vi "Main X-Y.vi"(0 "Home position X":dbl, 1 "Home position Y":dbl, 3 "Move position Y (# of steps)":dbl, 5 "Move position X (# of steps)":dbl, 7 "Change Home position Y?":bool, 9 "Return Home X":bool, 12 "Return Home Y":bool, 13 "Stop":bool, 14 "Move to Set Position":bool) -> (4 "Get/Acquire RT position X":dbl, 6 "Get/Acquire RT position Y":dbl, 8 "X-axes Motion":dbl(knob) scale=0.0..200.0, 10 "Y-axes Motion":dbl(knob) scale=0.0..200.0)   [LabVIEW 2018]
doc: "X-Y motion control simulator app that demonstrates control of the X-Y stage for a given system hardware"
panel:
  in  "Change Home position X?":bool
  out "System Ready?":bool
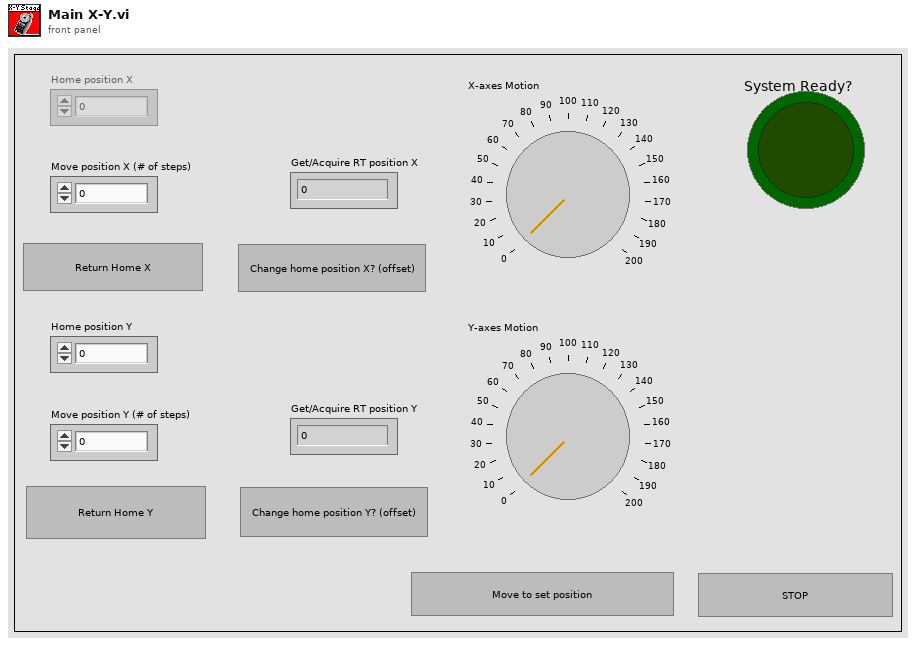
[diagram p1: front panel]
types:
  T1 = enum32{"Invalid", "Standard", "Closed", "Hidden", "Minimized", "Maximized"}
  T2 = enum32{"invalid app kind", "Development System", "Run Time System", "Student Edition", "Embedded LabVIEW", "Evaluation", "Custom"}
  T3 = enum8{"Enabled", "Disabled", "Disabled and Grayed Out"}
  T4 = cluster{"Core":cluster{"Current VI Reference":refnum<vi>, "Close Panel on Exit?":bool}, "System Ready?":bool, string}
  T5 = cluster{"Current VI Reference":refnum<vi>, "Close Panel on Exit?":bool}
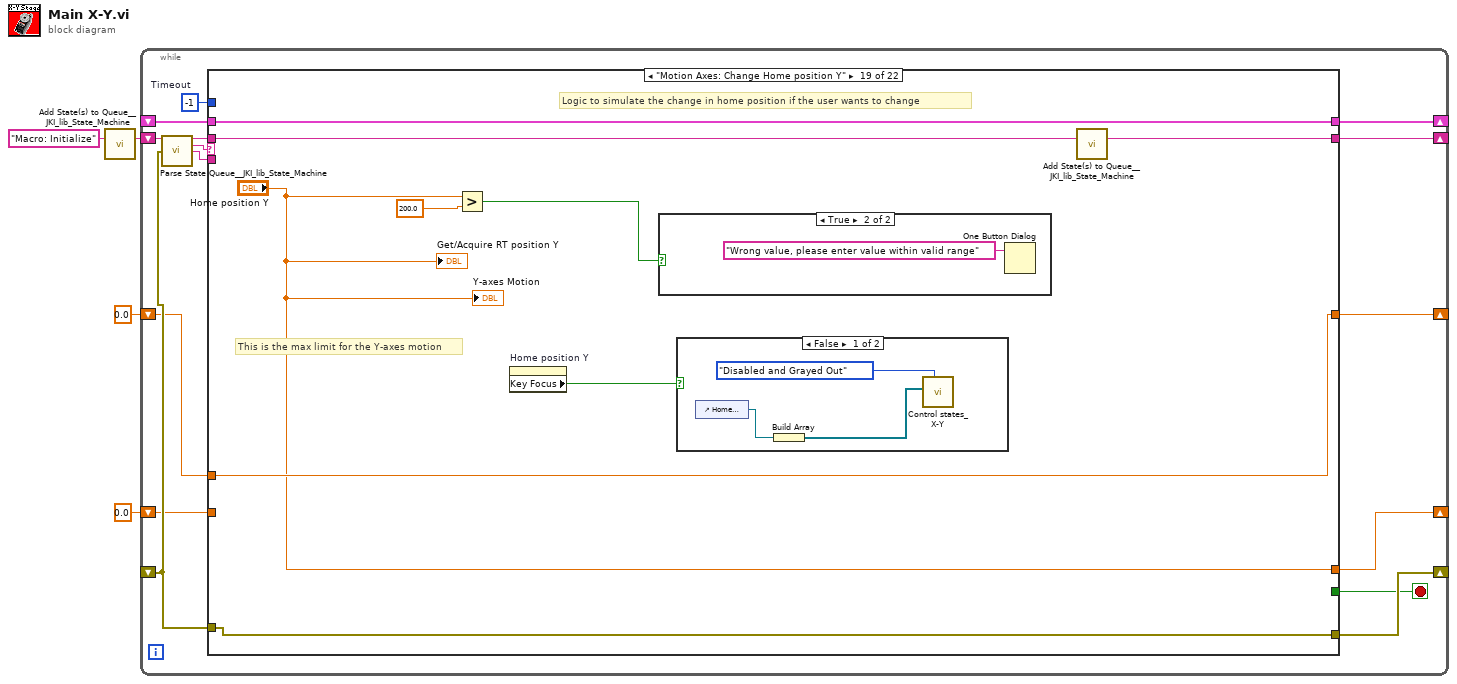
[diagram p0: block diagram]
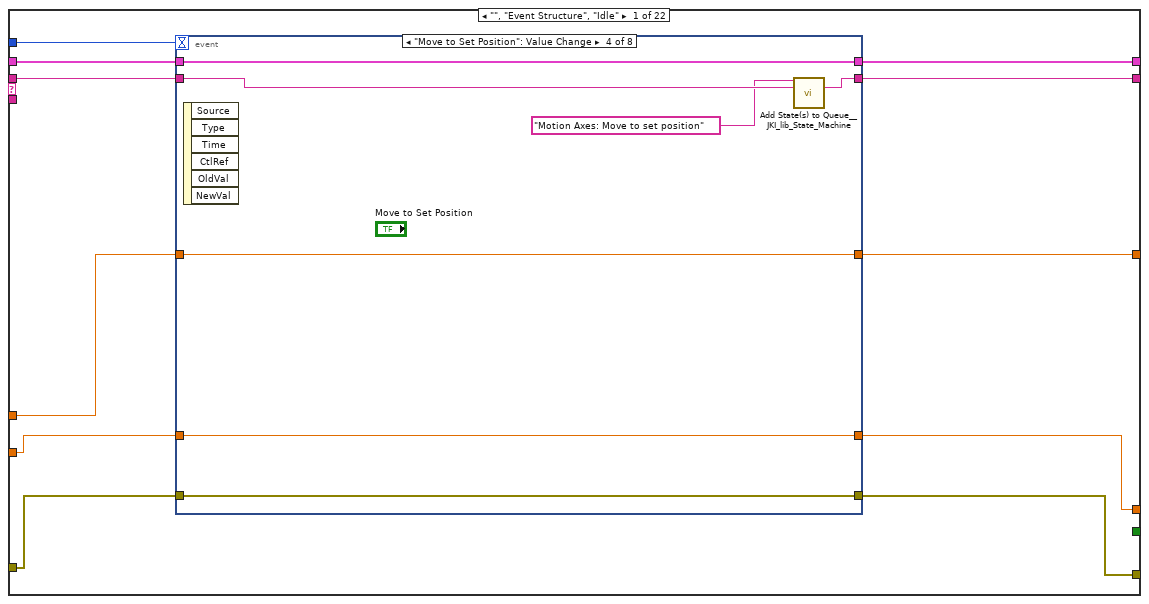
[diagram p2: hidden frame]
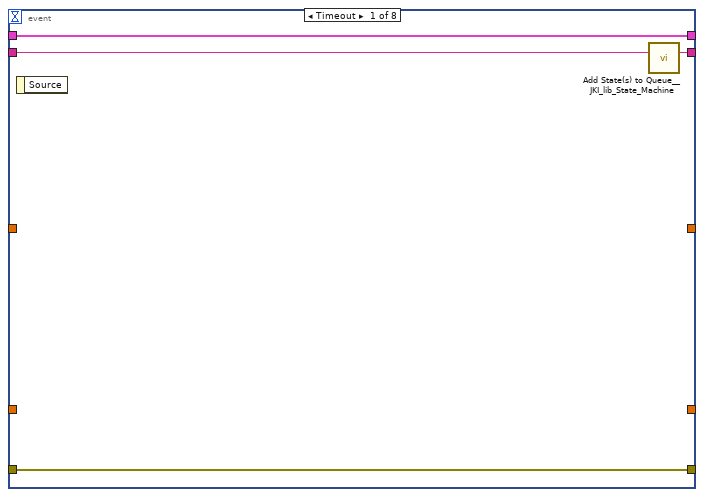
[diagram p3: hidden frame]
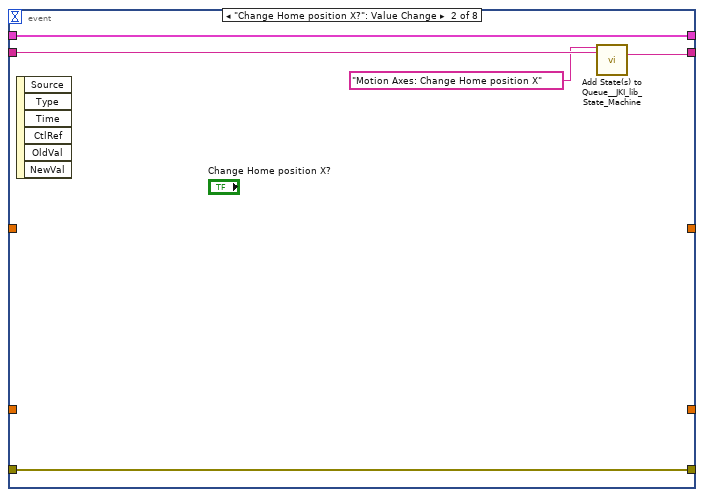
[diagram p4: hidden frame]
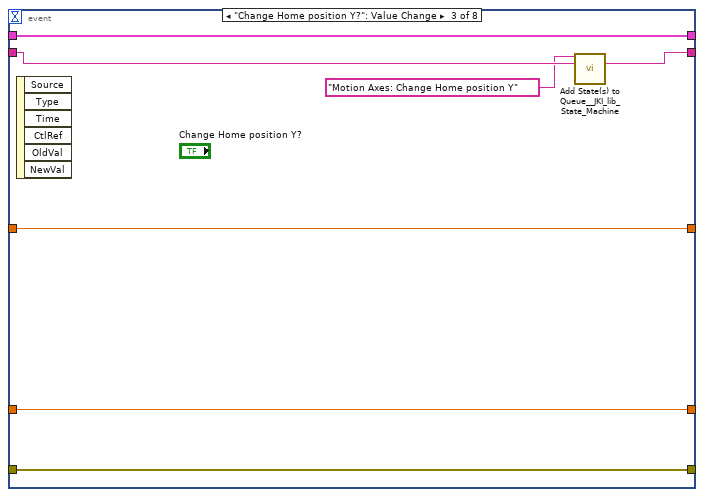
[diagram p5: hidden frame]
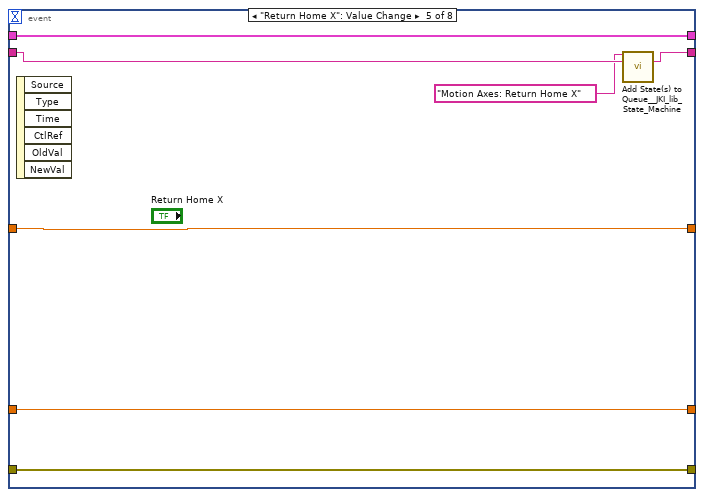
[diagram p6: hidden frame]
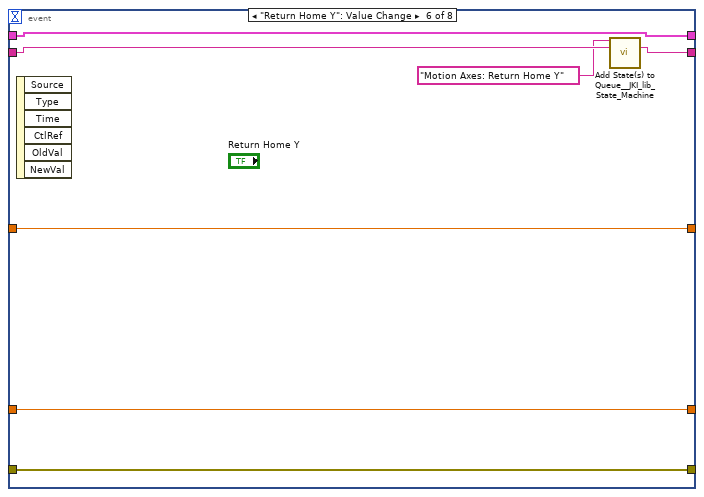
[diagram p7: hidden frame]
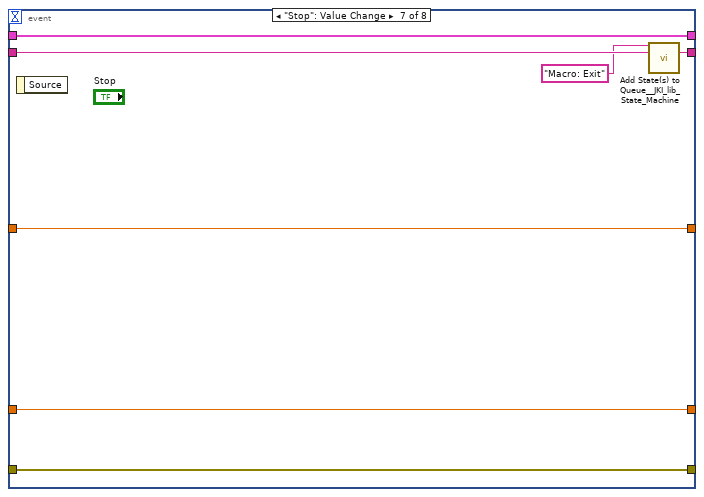
[diagram p8: hidden frame]
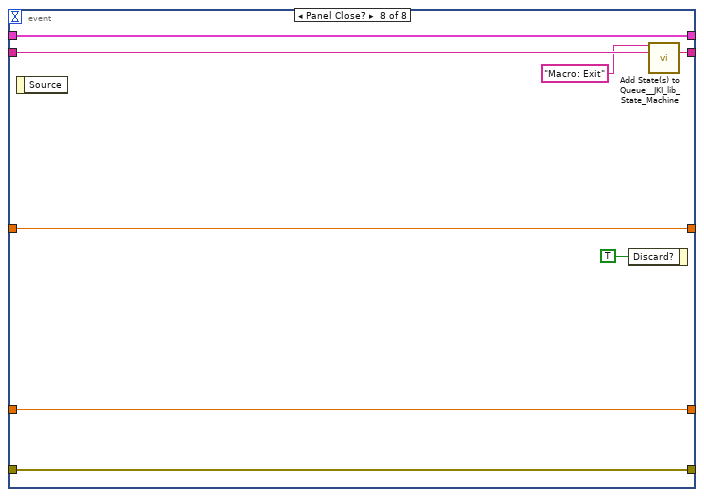
[diagram p9: hidden frame]
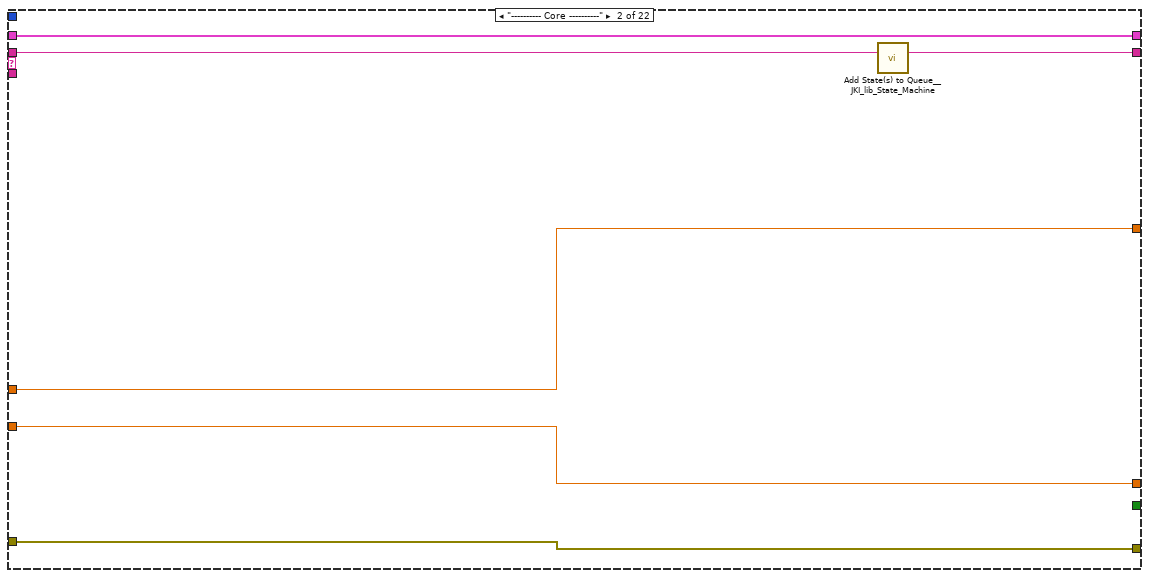
[diagram p10: hidden frame]
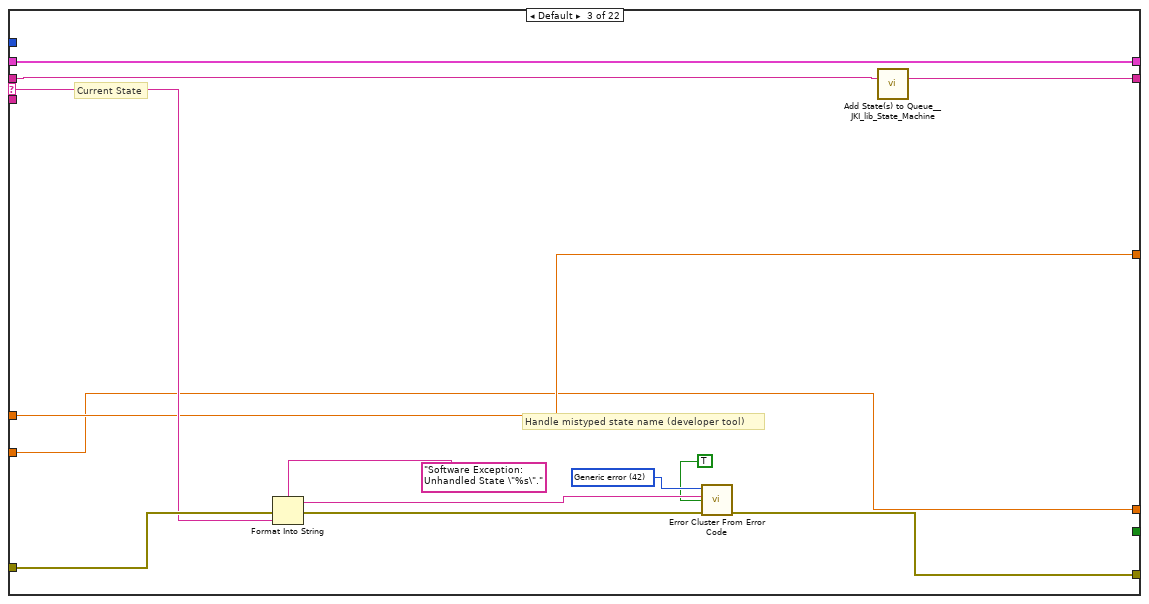
[diagram p11: hidden frame]
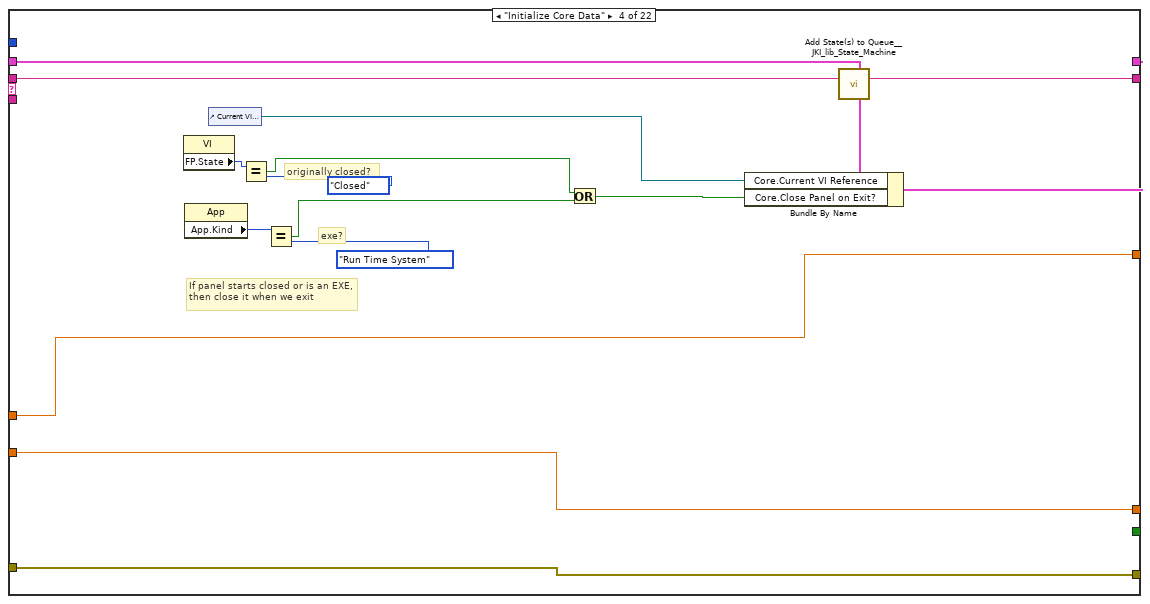
[diagram p12: hidden frame]
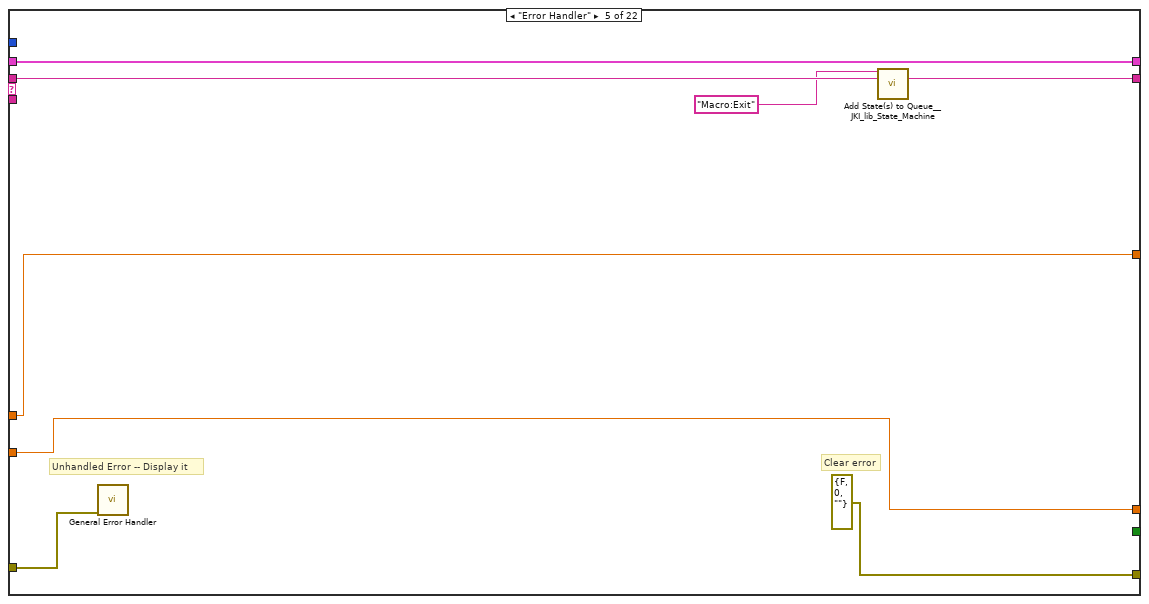
[diagram p13: hidden frame]
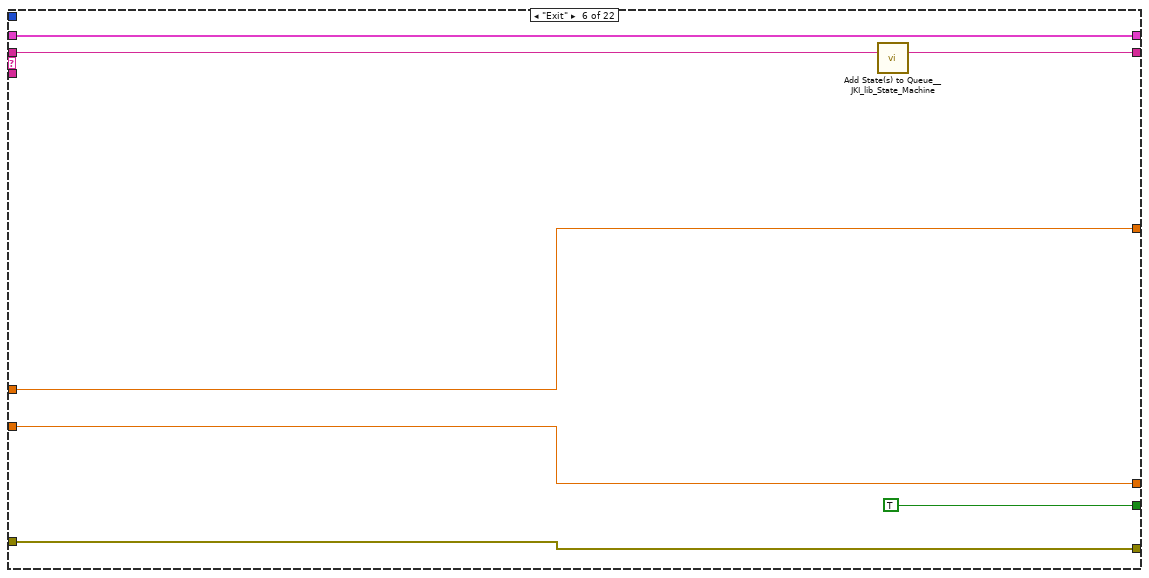
[diagram p14: hidden frame]
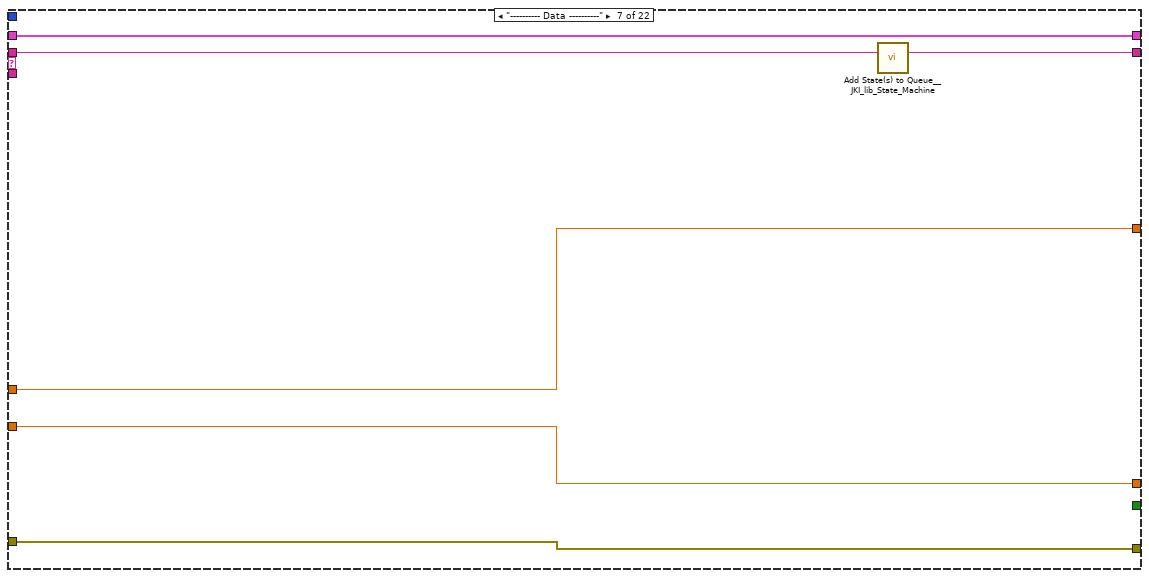
[diagram p15: hidden frame]
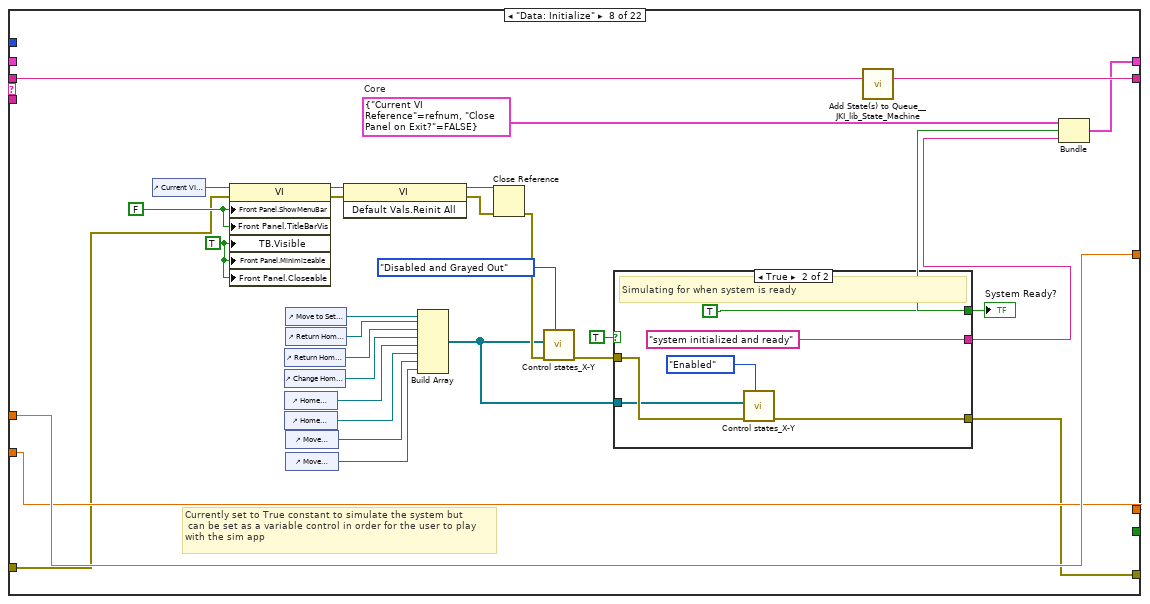
[diagram p16: hidden frame]
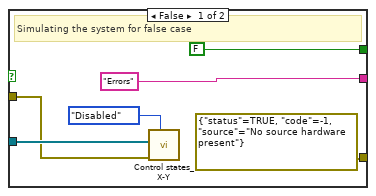
[diagram p17: hidden frame]
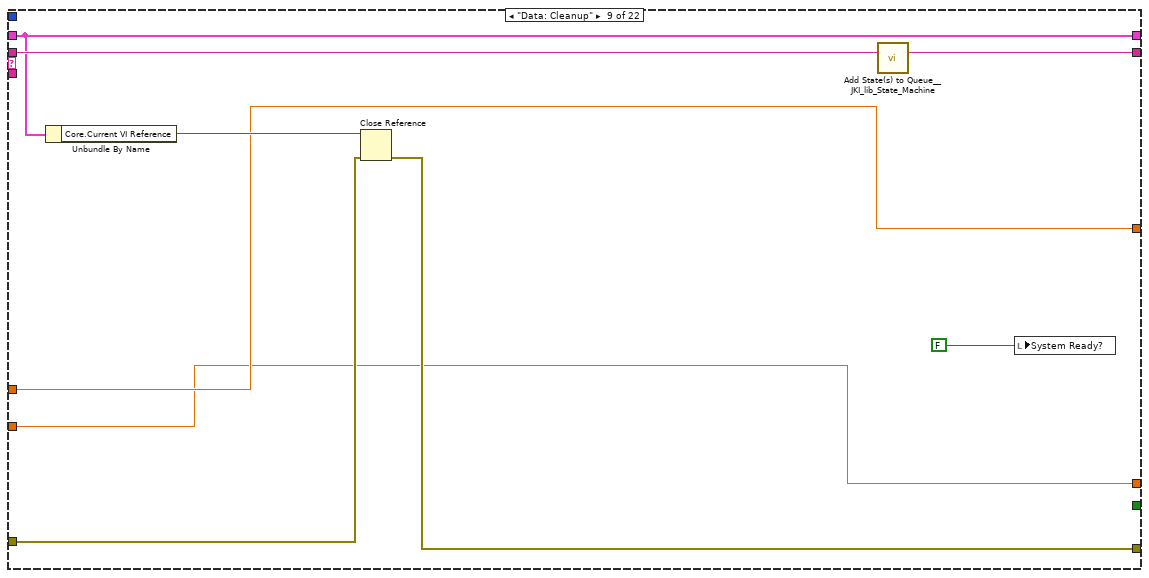
[diagram p18: hidden frame]
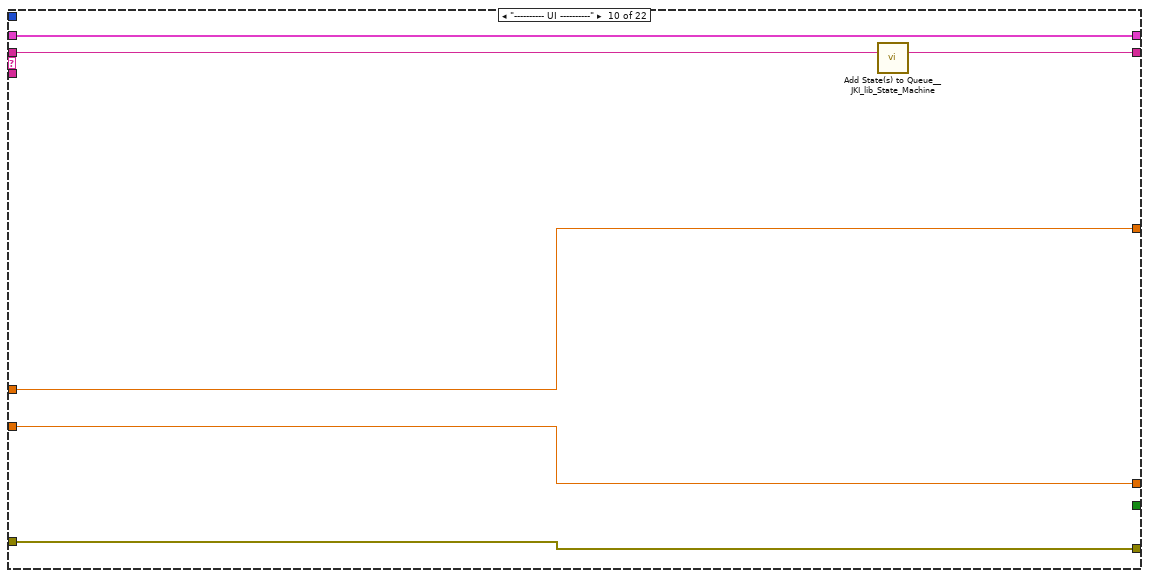
[diagram p19: hidden frame]
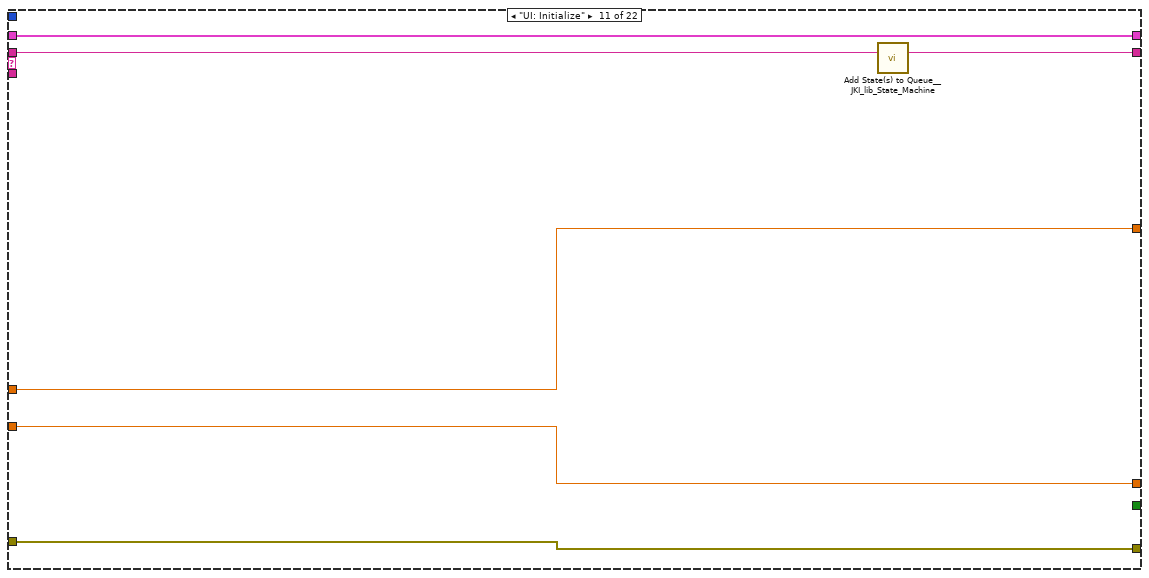
[diagram p20: hidden frame]
diagram:
  n1 = call <vilib>:"Add State(s) to Queue__JKI_lib_State_Machine.vi"("State(s) in (\"\")"="Macro: Initialize") -> ("States Out"=w4:string)  [unwired: 14 in]
  n2 = while "JKI State Machine 2018" {
    shift-right: [w12] -> _
    shift-left: _ -> [w11]
    shift-right: [w15] -> _
    shift-left: _ -> [w9]
    shift-right: [w14] -> _
    shift-left: w4 -> [w16]
    shift-right: [w8] -> _
    shift-left: 0.0 -> [w7]
    shift-right: [w6] -> _
    shift-left: 0.0 -> [w5]
    stop <- w13 stop-if-true
    w10 = -1  # Timeout
    n3 = call <vilib>:"Parse State Queue__JKI_lib_State_Machine.vi"("State Queue"=w16, "Error In (no error)"=w9) -> ("Remaining States"=w18:string, "Current State"=w19:string, "Arguments"=w17:string)  [unwired: 11 in]
    n4 = case shown="\"Motion Axes: Change Home position Y\"" w19 {
      selector: w19 -> [_ _ w91 _ _ _ _ _ _ _ _ _ _ _ _ _ _ _ _ _ _ _]
      tunnel: w18 -> [w30 w88 w95 w116 w124 w131 w137 w167 w188 w194 w200 w208 w221 w292 w299 w311 w317 w326 w339 w361 w373 w389]
      tunnel: w17 -> [_ _ _ _ _ _ _ _ _ _ _ w203 w215 _ _ _ _ _ _ _ _ _]
      tunnel: w11 -> [w28 w85 w93 w109 w121 w129 w134 _ w183 w191 w198 w206 w217 w289 w296 w308 w314 w324 w337 w358 w370 w386]
      tunnel: [w27 w86 w97 w113 errorcluster {"status"=FALSE, "code"=0, "source"=""} ("error out") w128 w135 w140 w184 w192 w197 w204 w218 w290 w297 w309 w315 w320 w334 w359 w371 w387] -> w15
      tunnel: w9 -> [w26 w86 w96 w113 w120 w128 w135 w154 w185 w192 w197 w205 w219 w290 w297 w309 w315 w320 w334 w359 w371 w387]
      tunnel: [w29 w87 w94 w115 w123 w130 w136 w166 w187 w193 w199 w207 w220 w291 w298 w310 w316 w325 w338 w360 w372 w388] -> w14
      tunnel: [_ _ _ _ _ TRUE _ _ _ _ _ _ _ _ _ _ _ _ _ _ _ _] -> w13
      tunnel: [w25 w85 w93 w114 w121 w129 w134 w165 w183 w191 w198 w206 w217 w289 w296 w308 w314 w324 w337 w358 w370 w386] -> w12
      tunnel: w10 -> [w24 _ _ _ _ _ _ _ _ _ _ _ _ _ _ _ _ _ _ _ _ _]
      tunnel: [w23 w84 w90 w103 w118 w126 w133 w163 w182 w190 w196 w202 w214 w288 w294 w301 w313 "Home position X" w333 w345 w366 w383] -> w8
      tunnel: w7 -> [w22 w84 w90 w103 w118 w126 w133 w163 w182 w190 w196 w202 w214 w288 w294 w301 w313 _ w333 w356 w365 w383]
      tunnel: [w21 w83 w89 w102 w117 w125 w132 w162 w181 w189 w195 w201 w213 w287 w293 w300 w312 w319 "Home position Y" w344 w367 w382] -> w6
      tunnel: w5 -> [w20 w83 w89 w102 w117 w125 w132 w162 w181 w189 w195 w201 w213 w287 w293 w300 w312 w319 _ w354 w367 w381]
      frame "", "Event Structure", "Idle" {
        n5 = event shown="[3] \"Move to Set Position\": Value Change" {
          selector: _ -> [_ _ _ _ _ _ _ _]
          dyn-events: _ -> [_ _ _ _ _ _ _ _]
          timeout: w24 -> [_ _ _ _ _ _ _ _]
          tunnel: w30 -> [w34 w38 w45 w52 w59 w67 w74 w82]
          tunnel: [w33 w37 w44 w50 w58 w61 w73 w81] -> w29
          tunnel: w28 -> [w31 w39 w46 w53 w60 w66 w71 w79]
          tunnel: [w32 w35 w42 w49 w56 w63 w72 w80] -> w27
          tunnel: w26 -> [w32 w35 w42 w49 w56 w63 w72 w80]
          tunnel: [w31 w39 w46 w53 w60 w66 w71 w79] -> w25
          tunnel: [_ _ w40 w48 w55 w65 w69 w76] -> w23
          tunnel: w22 -> [_ _ w40 w48 w55 w65 w69 w76]
          tunnel: [_ _ w41 w47 w54 w64 w68 w75] -> w21
          tunnel: w20 -> [_ _ w41 w47 w54 w64 w68 w75]
          event Timeout {
            n6 = event-data() -> ()  [unwired: 1 in, 1 out]
            n7 = call <vilib>:"Add State(s) to Queue__JKI_lib_State_Machine.vi"("State(s) in (\"\")"=w34) -> ("States Out"=w33:string)  [unwired: 14 in]
          }
          event "Change Home position X?": Value Change {
            n8 = event-data() -> ()  [unwired: 1 in, 6 out]
            n9 = call <vilib>:"Add State(s) to Queue__JKI_lib_State_Machine.vi"("State(s) in Front (\"\")"="Motion Axes: Change Home position X" ("State(s) in Front (\"\")"), "State(s) in (\"\")"=w38) -> ("States Out"=w37:string)  [unwired: 13 in]
          }
          event "Change Home position Y?": Value Change {
            n10 = event-data() -> ()  [unwired: 1 in, 6 out]
            n11 = call <vilib>:"Add State(s) to Queue__JKI_lib_State_Machine.vi"("State(s) in Front (\"\")"="Motion Axes: Change Home position Y" ("State(s) in Front (\"\")"), "State(s) in (\"\")"=w45) -> ("States Out"=w44:string)  [unwired: 13 in]
          }
          event "Move to Set Position": Value Change {
            n12 = event-data() -> ()  [unwired: 1 in, 6 out]
            n13 = call <vilib>:"Add State(s) to Queue__JKI_lib_State_Machine.vi"("State(s) in Front (\"\")"="Motion Axes: Move to set position" ("State(s) in Front (\"\")"), "State(s) in (\"\")"=w52) -> ("States Out"=w50:string)  [unwired: 13 in]
          }
          event "Return Home X": Value Change {
            n14 = event-data() -> ()  [unwired: 1 in, 6 out]
            n15 = call <vilib>:"Add State(s) to Queue__JKI_lib_State_Machine.vi"("State(s) in Front (\"\")"="Motion Axes: Return Home X" ("State(s) in Front (\"\")"), "State(s) in (\"\")"=w59) -> ("States Out"=w58:string)  [unwired: 13 in]
          }
          event "Return Home Y": Value Change {
            n16 = event-data() -> ()  [unwired: 1 in, 6 out]
            n17 = call <vilib>:"Add State(s) to Queue__JKI_lib_State_Machine.vi"("State(s) in Front (\"\")"="Motion Axes: Return Home Y" ("State(s) in Front (\"\")"), "State(s) in (\"\")"=w67) -> ("States Out"=w61:string)  [unwired: 13 in]
          }
          event "Stop": Value Change {
            n18 = event-data() -> ()  [unwired: 1 in, 1 out]
            n19 = call <vilib>:"Add State(s) to Queue__JKI_lib_State_Machine.vi"("State(s) in Front (\"\")"="Macro: Exit", "State(s) in (\"\")"=w74) -> ("States Out"=w73:string)  [unwired: 13 in]
          }
          event Panel Close? {
            n20 = event-data() -> ()  [unwired: 1 in, 1 out]
            n21 = event-data("Discard?"=TRUE) -> ()  [unwired: 1 in, 1 out]
            n22 = call <vilib>:"Add State(s) to Queue__JKI_lib_State_Machine.vi"("State(s) in Front (\"\")"="Macro: Exit", "State(s) in (\"\")"=w82) -> ("States Out"=w81:string)  [unwired: 13 in]
          }
        }
      }
      frame "---------- Core ----------" {
        n23 = call <vilib>:"Add State(s) to Queue__JKI_lib_State_Machine.vi"("State(s) in (\"\")"=w88) -> ("States Out"=w87:string)  [unwired: 14 in]
      }
      frame Default {
        w100 = 42 items=["No error", "Argument error", "Memory is full", "Out of zone", "End of file", "File already open", "Generic file I/O error", "File not found", "File permission error", "Disk is full", "Duplicate path", "Too many files open", "System feature not enabled", "Resource file not found", "Cannot add resource", "Resource not found", "Image not found", "Image memory error", "Pen does not exist", "Config type invalid", "Config token not found", "Config parse error", "Config memory error", "Bad external code format", "Bad external code offset", "External code not present", "Null window", "Destroy window error", "Null menu", "Print aborted", "Bad print record", "Print driver error", "Windows error during printing", "Memory error during printing", "Print dialog error", "Generic print error", "Invalid device refnum", "Device not found", "Device parameter error", "Device unit error", "Cannot open device", "Device call aborted", "Generic error", "Cancelled by user", "Object ID too low", "Object ID too high", "Object not in heap", "Unknown heap", "Unknown object (invalid DefProc)", "Unknown object (DefProc not in table)", "Message out of range", "Invalid (null) method", "Unknown message", "Manager call not supported", "Bad address", "Network operation in progress", "Network operation timed out", "Connection is busy", "Network attribute not supported", "Network error", "Address in use", "System out of memory", "Connection aborted", "Connection refused", "Not connected", "Already connected", "Connection closed", "Initialization error (interapplication manager)", "Bad occurrence", "Wait on unbound occurrence handler", "Occurrence queue overflow", "Datalog type conflict", "Unused", "Unrecognized type (interapplication manager)", "Memory corrupt", "Failed to make temporary DLL", "Old CIN version", "Drag socket not found", "Failed to load drop-object", "Failed to register OLE object", "Failed to release OLE object", "Format specifier type mismatch", "Unknown format specifier", "Too few format specifiers", "Too many format specifiers", "Scan failed", "Newer CIN version", "Error converting to variant", "Runtime menu error", "Password tampered", "Variant attribute not found", "Incompatible variant data type", "Event data is not available", "Event Store is not present", "Occurrence is not found", "Event Queue is not created", "Event info is not available", "Refnum passed is NULL", "Error retrieving Class GUID", "Error retrieving CoClass GUID", "Error retrieving TypeLib GUID.", "Bad built application magic bytes.", "Specific driver is different from the specific driver associated with the Logical Name.", "There is no session opened to the class driver.", "Max Error", "MAX - Error with config objects", "MAX - Error loading configuration", "MAX - Group not supported"]
        # "Current State"
        # "Handle mistyped state name (developer tool)"
        n24 = Format Into String(format string="Software Exception: Unhandled State \"%s\"." ("message"), error in=w96, w91) -> (resulting string=w99:string, error out=w98:errorcluster)  [unwired: 1 in]
        n25 = call <vilib>:"Error Cluster From Error Code.vi"("show call chain? (False)"=TRUE, "error in (no error)"=w98, "error message (\"\")"=w99, "error code (0)"=w100) -> ("error out"=w97:errorcluster)  [unwired: 5 in]
        n26 = call <vilib>:"Add State(s) to Queue__JKI_lib_State_Machine.vi"("State(s) in (\"\")"=w95) -> ("States Out"=w94:string)  [unwired: 14 in]
      }
      frame "Initialize Core Data" {
        # "originally closed?"
        # "exe?"
        # "If panel starts closed or is an EXE, then close it when we exit"
        n27 = property class="VI"() -> ("FP.State"=w106:T1)  [unwired: 2 in, 2 out]
        n28 = property class="App"() -> ("App.Kind"=w112:T2)  [unwired: 2 in, 2 out]
        n29 = control-ref of="Current VI Reference"() -> (w107:refnum<vi>)
        n30 = Equal?(x=w106, y=T1."Closed" ("Front Panel Window:State")) -> (x = y?=w104:bool)
        n31 = Equal?(x=w112, y=T2."Run Time System" ("Application:Kind")) -> (x = y?=w110:bool)
        n32 = Or(x=w104, y=w110) -> (x .or. y?=w108:bool)
        n33 = Bundle By Name(cluster=w109, "Core.Current VI Reference"=w107, "Core.Close Panel on Exit?"=w108) -> (w114:T4)
        n34 = call <vilib>:"Add State(s) to Queue__JKI_lib_State_Machine.vi"("State(s) in (\"\")"=w116) -> ("States Out"=w115:string)  [unwired: 14 in]
      }
      frame "Error Handler" {
        # "Unhandled Error -- Display it"
        # "Clear error"
        n35 = call <vilib>:"General Error Handler.vi"("error in (no error)"=w120) -> ()  [unwired: 10 in, 5 out]
        n36 = call <vilib>:"Add State(s) to Queue__JKI_lib_State_Machine.vi"("State(s) in Front (\"\")"="Macro:Exit", "State(s) in (\"\")"=w124) -> ("States Out"=w123:string)  [unwired: 13 in]
      }
      frame "Exit" {
        n37 = call <vilib>:"Add State(s) to Queue__JKI_lib_State_Machine.vi"("State(s) in (\"\")"=w131) -> ("States Out"=w130:string)  [unwired: 14 in]
      }
      frame "---------- Data ----------" {
        n38 = call <vilib>:"Add State(s) to Queue__JKI_lib_State_Machine.vi"("State(s) in (\"\")"=w137) -> ("States Out"=w136:string)  [unwired: 14 in]
      }
      frame "Data: Initialize" {
        w159 = TRUE ("Tool Bar:Visible")
        w160 = FALSE ("Front Panel Window:Show Menu Bar")
        w164 = T5 {"Current VI Reference"=refnum, "Close Panel on Exit?"=FALSE}  # Core
        # "Currently set to True constant to simulate the system but\n can be set as a variable control in order for the user to play\nwith the sim app"
        n39 = control-ref of="Current VI Reference"() -> (w161:refnum<vi>)
        n40 = property class="VI"(reference=w161, error in=w154, "Front Panel.ShowMenuBar"=w160, "Front Panel.TitleBarVis"=w160, "TB.Visible"=w159, "Front Panel.Minimizeable"=w159, "Front Panel.Closeable"=w159) -> (reference out=w158:refnum<vi>, error out=w157:errorcluster)
        n41 = control-ref of="Return Home X"() -> (w151:refnum<vi>)
        n42 = control-ref of="Change Home position Y?"() -> (w150:refnum<vi>)
        n43 = control-ref of="Home position X"() -> (w149:refnum<vi>)
        n44 = control-ref of="Home position Y"() -> (w148:refnum<vi>)
        n45 = control-ref of="Move to Set Position"() -> (w153:refnum<vi>)
        n46 = control-ref of="Return Home Y"() -> (w152:refnum<vi>)
        n47 = control-ref of="Move position Y (# of steps)"() -> (w147:refnum<vi>)
        n48 = control-ref of="Move position X (# of steps)"() -> (w146:refnum<vi>)
        n49 = invoke class="VI" method="Default Vals.Reinit All"(reference=w158, error in=w157) -> (reference out=w156:refnum<vi>, error out=w155:errorcluster)  [unwired: 1 in, 1 out]
        n50 = Build Array(w153, w152, w151, w150, w149, w148, w147, w146) -> (w141:refnum<vi>[])
        n51 = Close Reference(reference=w156, error in (no error)=w155) -> (error out=w145:errorcluster)
        n52 = call "Control states_X-Y.vi"("Command"=T3."Disabled and Grayed Out", "error in (no error)"=w145, "Reference in"=w141) -> ("error out"=w142:errorcluster)  [unwired: 8 in]
        n53 = case shown="True" TRUE {
          tunnel: w142 -> [w170 w177]
          tunnel: ["Errors" "system initialized and ready"] -> w139
          tunnel: [FALSE ("System Ready?") TRUE ("System Ready?")] -> w138
          tunnel: w141 -> [w171 w176]
          tunnel: [errorcluster {"status"=TRUE, "code"=-1, "source"="No source hardware present"} ("error out") w174] -> w140
          frame False {
            # "Simulating the system for false case"
            n54 = call "Control states_X-Y.vi"("Command"=T3."Disabled", "error in (no error)"=w170, "Reference in"=w171) -> ()  [unwired: 8 in, 1 out]
          }
          frame True {
            # "Simulating for when system is ready"
            n55 = call "Control states_X-Y.vi"("Command"=T3."Enabled", "error in (no error)"=w177, "Reference in"=w176) -> ("error out"=w174:errorcluster)  [unwired: 8 in]
          }
        }
        "System Ready?" <- w138
        n56 = call <vilib>:"Add State(s) to Queue__JKI_lib_State_Machine.vi"("State(s) in (\"\")"=w167) -> ("States Out"=w166:string)  [unwired: 14 in]
        n57 = Bundle("Core"=w164, "System Ready?"=w138, w139) -> (w165:T4)  [unwired: 1 in]
      }
      frame "Data: Cleanup" {
        n58 = Unbundle By Name(w183) -> ("Core.Current VI Reference"=w186:refnum<vi>)
        n59 = Close Reference(reference=w186, error in (no error)=w185) -> (error out=w184:errorcluster)
        n60 = call <vilib>:"Add State(s) to Queue__JKI_lib_State_Machine.vi"("State(s) in (\"\")"=w188) -> ("States Out"=w187:string)  [unwired: 14 in]
        n61 = local write "System Ready?"(FALSE ("System Ready?")) -> ()
      }
      frame "---------- UI ----------" {
        n62 = call <vilib>:"Add State(s) to Queue__JKI_lib_State_Machine.vi"("State(s) in (\"\")"=w194) -> ("States Out"=w193:string)  [unwired: 14 in]
      }
      frame "UI: Initialize" {
        n63 = call <vilib>:"Add State(s) to Queue__JKI_lib_State_Machine.vi"("State(s) in (\"\")"=w200) -> ("States Out"=w199:string)  [unwired: 14 in]
      }
      frame "UI: Cursor Set" {
        # "Argument"
        n64 = case shown="\"Idle\", Default" w203 {
          tunnel: w205 -> [w210 w212]
          tunnel: [w209 w211] -> w204
          frame "Idle", Default {
            n65 = call <vilib>:"Unset Busy.vi"("error in (no error)"=w210) -> ("error out"=w209:errorcluster)  [unwired: 10 in]
          }
          frame "Busy" {
            n66 = call <vilib>:"Set Busy.vi"("error in (no error)"=w212) -> ("error out"=w211:errorcluster)  [unwired: 9 in, 1 out]
          }
        }
        n67 = call <vilib>:"Add State(s) to Queue__JKI_lib_State_Machine.vi"("State(s) in (\"\")"=w208) -> ("States Out"=w207:string)  [unwired: 14 in]
      }
      frame "UI: Front Panel State" {
        # "Argument"
        n68 = Unbundle By Name(w217) -> ("Core.Current VI Reference"=w216:refnum<vi>)
        n69 = case shown="\"Hidden\", \"Hide\"" w215 {
          tunnel: w219 -> [w227 w242 w253 w266 w279]
          tunnel: [w229 w243 w255 w268 w281] -> w218
          tunnel: w216 -> [w228 w240 w254 w267 w280]
          frame "Open", "Standard", Default {
            w222 = T1."Standard" ("State")
            n70 = property class="VI"(reference=w228, error in=w227) -> (reference out=w225:refnum<vi>, error out=w226:errorcluster, "FP.State"=w224:T1)
            n71 = Not Equal?(x=w224, y=w222) -> (x != y?=w223:bool)
            n72 = case shown="True" w223 {
              tunnel: [w233 w235] -> w229
              tunnel: w226 -> [w232 w235]
              tunnel: w225 -> [w231 _]
              tunnel: w222 -> [w230 _]
              frame True {
                n73 = invoke class="VI" method="FP.Open"(reference=w231, error in=w232, "Activate"=TRUE, "State"=w230) -> (error out=w233:errorcluster)  [unwired: 1 in, 4 out]
              }
              frame False {
              }
            }
          }
          frame "Close", "Closed" {
            n74 = property class="VI"(reference=w240, error in=w242) -> (reference out=w239:refnum<vi>, error out=w241:errorcluster, "FP.State"=w237:T1)
            n75 = Not Equal?(x=w237, y=T1."Closed" ("Front Panel Window:State")) -> (x != y?=w236:bool)
            n76 = case shown="True" w236 {
              tunnel: [w244 w247] -> w243
              tunnel: w241 -> [w244 w246]
              tunnel: w239 -> [_ w245]
              frame False {
              }
              frame True {
                n77 = invoke class="VI" method="FP.Close"(reference=w245, error in=w246) -> (error out=w247:errorcluster)  [unwired: 1 in, 2 out]
              }
            }
          }
          frame "Hidden", "Hide" {
            w248 = T1."Hidden" ("State")
            n78 = property class="VI"(reference=w254, error in=w253) -> (reference out=w251:refnum<vi>, error out=w252:errorcluster, "FP.State"=w250:T1)
            n79 = Not Equal?(x=w250, y=w248) -> (x != y?=w249:bool)
            n80 = case shown="True" w249 {
              tunnel: [w259 w260] -> w255
              tunnel: w252 -> [w258 w260]
              tunnel: w251 -> [w257 _]
              tunnel: w248 -> [w256 _]
              frame True {
                n81 = invoke class="VI" method="FP.Open"(reference=w257, error in=w258, "State"=w256) -> (error out=w259:errorcluster)  [unwired: 2 in, 4 out]
              }
              frame False {
              }
            }
          }
          frame "Minimize", "Minimized" {
            w261 = T1."Minimized" ("State")
            n82 = property class="VI"(reference=w267, error in=w266) -> (reference out=w264:refnum<vi>, error out=w265:errorcluster, "FP.State"=w263:T1)
            n83 = Not Equal?(x=w263, y=w261) -> (x != y?=w262:bool)
            n84 = case shown="True" w262 {
              tunnel: [w272 w273] -> w268
              tunnel: w265 -> [w271 w273]
              tunnel: w264 -> [w270 _]
              tunnel: w261 -> [w269 _]
              frame True {
                n85 = invoke class="VI" method="FP.Open"(reference=w270, error in=w271, "State"=w269) -> (error out=w272:errorcluster)  [unwired: 2 in, 4 out]
              }
              frame False {
              }
            }
          }
          frame "Maximize", "Maximized" {
            w274 = T1."Maximized" ("State")
            n86 = property class="VI"(reference=w280, error in=w279) -> (reference out=w277:refnum<vi>, error out=w278:errorcluster, "FP.State"=w276:T1)
            n87 = Not Equal?(x=w276, y=w274) -> (x != y?=w275:bool)
            n88 = case shown="True" w275 {
              tunnel: [w285 w286] -> w281
              tunnel: w278 -> [w284 w286]
              tunnel: w277 -> [w283 _]
              tunnel: w274 -> [w282 _]
              frame True {
                n89 = invoke class="VI" method="FP.Open"(reference=w283, error in=w284, "State"=w282) -> (error out=w285:errorcluster)  [unwired: 2 in, 4 out]
              }
              frame False {
              }
            }
          }
        }
        n90 = call <vilib>:"Add State(s) to Queue__JKI_lib_State_Machine.vi"("State(s) in (\"\")"=w221) -> ("States Out"=w220:string)  [unwired: 14 in]
      }
      frame "---------- Macro ----------" {
        n91 = call <vilib>:"Add State(s) to Queue__JKI_lib_State_Machine.vi"("State(s) in (\"\")"=w292) -> ("States Out"=w291:string)  [unwired: 14 in]
      }
      frame "Macro: Initialize" {
        w295 = "Data: Initialize\nInitialize Core Data\nUI: Initialize\nUI: Front Panel State >> Open"  # Data: Initialize Initialize Core Data UI: Initialize UI: Front Panel State >> Open
        n92 = call <vilib>:"Add State(s) to Queue__JKI_lib_State_Machine.vi"("State(s) in Front (\"\")"=w295, "State(s) in (\"\")"=w299) -> ("States Out"=w298:string)  [unwired: 13 in]
      }
      frame "Macro: Exit" {
        n93 = Unbundle By Name(w308) -> ("Core.Close Panel on Exit?"=w307:bool)
        n94 = Select(t="UI: Front Panel State >> Close", s=w307, f="") -> (s? t:f=w304:string)
        n95 = call <vilib>:"Add State(s) to Queue__JKI_lib_State_Machine.vi"("State(s) in (\"\")"=w304, "State(s) at Back (\"\")"="Data: Cleanup\nExit") -> ("States Out"=w302:string)  [unwired: 13 in]
        n96 = call <vilib>:"Add State(s) to Queue__JKI_lib_State_Machine.vi"("State(s) in Front (\"\")"=w302, "State(s) in (\"\")"=w311) -> ("States Out"=w310:string)  [unwired: 13 in]
      }
      frame "---------- Motion Axes ----------" {
        n97 = call <vilib>:"Add State(s) to Queue__JKI_lib_State_Machine.vi"("State(s) in (\"\")"=w317) -> ("States Out"=w316:string)  [unwired: 14 in]
      }
      frame "Motion Axes: Change Home position X" {
        # "This is the max limit for the X-axes motion"
        # "Logic to simulate the change in home position if the user wants to change"
        n98 = property on="Home position X" class="DigNum (strict)"() -> ("Key Focus"=w321:bool)  [unwired: 2 in, 2 out]
        n99 = Greater?(x="Home position X", y=200.0) -> (0:w322:bool)
        n100 = case shown="True" w322 {
          frame False {
          }
          frame True {
            n101 = One Button Dialog(message="Wrong value, please enter value within valid range") -> ()  [unwired: 1 in, 1 out]
          }
        }
        n102 = case shown="False" w321 {
          frame False {
            n103 = control-ref of="Home position X"() -> (w329:refnum<vi>)
            n104 = Build Array(w329) -> (w328:refnum<vi>[])
            n105 = call "Control states_X-Y.vi"("Command"=T3."Disabled and Grayed Out", "Reference in"=w328) -> ()  [unwired: 9 in, 1 out]
          }
          frame True {
          }
        }
        n106 = call <vilib>:"Add State(s) to Queue__JKI_lib_State_Machine.vi"("State(s) in (\"\")"=w326) -> ("States Out"=w325:string)  [unwired: 14 in]
        "Get/Acquire RT position X" <- "Home position X"
        "X-axes Motion" <- "Home position X"
      }
      frame "Motion Axes: Change Home position Y" {
        # "This is the max limit for the Y-axes motion"
        # "Logic to simulate the change in home position if the user wants to change"
        n107 = Greater?(x="Home position Y", y=200.0) -> (0:w335:bool)
        n108 = property on="Home position Y" class="DigNum (strict)"() -> ("Key Focus"=w331:bool)  [unwired: 2 in, 2 out]
        n109 = case shown="True" w335 {
          frame False {
          }
          frame True {
            n110 = One Button Dialog(message="Wrong value, please enter value within valid range") -> ()  [unwired: 1 in, 1 out]
          }
        }
        n111 = case shown="False" w331 {
          frame False {
            n112 = control-ref of="Home position Y"() -> (w340:refnum<vi>)
            n113 = Build Array(w340) -> (w342:refnum<vi>[])
            n114 = call "Control states_X-Y.vi"("Command"=T3."Disabled and Grayed Out", "Reference in"=w342) -> ()  [unwired: 9 in, 1 out]
          }
          frame True {
          }
        }
        n115 = call <vilib>:"Add State(s) to Queue__JKI_lib_State_Machine.vi"("State(s) in (\"\")"=w339) -> ("States Out"=w338:string)  [unwired: 14 in]
        "Get/Acquire RT position Y" <- "Home position Y"
        "Y-axes Motion" <- "Home position Y"
      }
      frame "Motion Axes: Move to set position" {
        # "Logic to simulate motion axes hardware movement"
        n116 = Add(x="Move position X (# of steps)", y=w356) -> (x+y=w350:dbl)
        n117 = Add(x="Move position Y (# of steps)", y=w354) -> (x+y=w348:dbl)
        n118 = Greater?(x=w350, y=200.0) -> (0:w347:bool)
        n119 = Greater?(x=w348, y=200.0) -> (0:w346:bool)
        n120 = Select(t=0.0, s=w347, f=w350) -> (s? t:f=w345:dbl)
        n121 = Select(t=0.0, s=w346, f=w348) -> (s? t:f=w344:dbl)
        n122 = local write "X-axes Motion"(w345) -> ()
        n123 = local write "Get/Acquire RT position X"(w345) -> ()
        n124 = local write "Y-axes Motion"(w344) -> ()
        n125 = local write "Get/Acquire RT position Y"(w344) -> ()
        n126 = case shown="True" w346 {
          frame False {
          }
          frame True {
            n127 = One Button Dialog(message="Position resets, please enter value within valid range") -> ()  [unwired: 1 in, 1 out]
          }
        }
        n128 = case shown="True" w347 {
          frame False {
          }
          frame True {
            n129 = One Button Dialog(message="Position resets, please enter value within valid range") -> ()  [unwired: 1 in, 1 out]
          }
        }
        n130 = call <vilib>:"Add State(s) to Queue__JKI_lib_State_Machine.vi"("State(s) in (\"\")"=w361) -> ("States Out"=w360:string)  [unwired: 14 in]
      }
      frame "Motion Axes: Return Home X" {
        # "Motion axes homing routine, rotates counter clockwise to return back"
        n131 = local read "Get/Acquire RT position X"() -> (w369:dbl)
        n132 = local read "Home position X"() -> (w364:dbl)
        n133 = Equal?(x=w364, y=w369) -> (x = y?=w368:bool)
        n134 = case shown="False" w368 {
          tunnel: [w376 w379] -> w366
          tunnel: w365 -> [_ w379]
          frame False {
            n135 = local read "Get/Acquire RT position X"() -> (w377:dbl)
            n136 = local read "Home position X"() -> (w378:dbl)
            n137 = Subtract(x=w377, y=w378) -> (x-y=w374:dbl)
            n138 = Negate(x=w374) -> (-x=w375:dbl)
            n139 = Add(x=w375, y=w377) -> (x+y=w376:dbl)
            n140 = local write "X-axes Motion"(w376) -> ()
            n141 = local write "Get/Acquire RT position X"(w376) -> ()
          }
          frame True {
          }
        }
        n142 = call <vilib>:"Add State(s) to Queue__JKI_lib_State_Machine.vi"("State(s) in (\"\")"=w373) -> ("States Out"=w372:string)  [unwired: 14 in]
      }
      frame "Motion Axes: Return Home Y" {
        # "Motion axes homing routine, rotates counter clockwise to return back"
        n143 = local read "Get/Acquire RT position Y"() -> (w385:dbl)
        n144 = local read "Home position Y"() -> (w380:dbl)
        n145 = Equal?(x=w380, y=w385) -> (x = y?=w384:bool)
        n146 = case shown="False" w384 {
          tunnel: [w392 w396] -> w382
          tunnel: w381 -> [_ w396]
          frame False {
            n147 = local read "Get/Acquire RT position Y"() -> (w395:dbl)
            n148 = local read "Home position Y"() -> (w394:dbl)
            n149 = local read "Get/Acquire RT position Y"() -> (w393:dbl)
            n150 = Subtract(x=w395, y=w394) -> (x-y=w391:dbl)
            n151 = Negate(x=w391) -> (-x=w390:dbl)
            n152 = Add(x=w390, y=w393) -> (x+y=w392:dbl)
            n153 = local write "Get/Acquire RT position Y"(w392) -> ()
            n154 = local write "Y-axes Motion"(w392) -> ()
          }
          frame True {
          }
        }
        n155 = call <vilib>:"Add State(s) to Queue__JKI_lib_State_Machine.vi"("State(s) in (\"\")"=w389) -> ("States Out"=w388:string)  [unwired: 14 in]
      }
    }
  }
